vi "PR_Recording_post-processing.vi"(7 "Progress Bar Dialog in":refnum<class "Progress Bar Dialog.lvclass">, 8 "error in (no error)":errorcluster, 9 "Processing parameters":T2={"Defragment TDMS? (F)"=FALSE, "Start time (SW)"=timestamp(0 s since 1904-01-01), "Start time (HW)"=0, "Data filtering"={"Filter type"=enum."Savitzky-Golay", "Length"=41, "Order"=3}, "Mouse drawing parameters"={"Trace length, samples"=0, "Rainbow track"=FALSE, "Rainbow track is speed"=FALSE, "Bright mouse lineout"=FALSE, "Colors array"=[], "Pixels per mm"=0.0}, "Size of the image (480x480)"={"Numeric Control"=480.0, "Numeric Control"=480.0}, "Image ref. in"=refnum, "Calibration parameters"={"Timing calibration sw/hw"=1.0, "True FPS"=80.0, "True frame time, s"=0.0125, "Disp. calibration info"=[]}, "Pixel to zone"=[]} {"Calibration parameters"."True frame time, s" format="%.10g"; "Calibration parameters"."Disp. calibration info"."Speed, µl per ms" format="%.3g"; "Calibration parameters"."True FPS" format="%.10g"; "Calibration parameters"."Timing calibration sw/hw" format="%.10g"; "Data filtering"."Order" min=3 max=11 step=2; "Data filtering"."Length" min=5 max=301 step=2}, 10 "Paths":T9, 11 "Settings cluster":T10={"Defaults"={"Default User"=0.0, "VISA Resource Name "="", "Histogram parameters"={"max"=300.0, "min"=0.0, "# bins"=10, "threshold"=8.0, "thr. type"=enum."higher accepted"}}, "Recording and saving"={"Researcher name"="", "Name prefix"="", "Data post-processing"={"Filter type"=enum."None", "Length"=0, "Order"=0}, "Stop at"=0.0, "\"Stop at\" enabled"=FALSE, "Default save folder path"=path "", "Acquisition FPS"=enum."Max"}, "Geometry"={"Cage diameter, mm"=0, "Starting angle MIDFIELD"=0, "Starting angle BORDER"=0, "Radius, mm CENTER"=0, "Radius, mm MIDFIELD"=0, "N segments MIDFIELD"=0, "N segments BORDER"=0, "R-gap, mm"=0.0, "Bridge swap"=FALSE, "Bridge H. offset"=0.0, "Bridge V. offset"=0.0, "Twisted neck"=FALSE, "Alt. magn. orientation"=FALSE, "Sensor board size"=enum."Small"}, "IO parameters"={"IO general config."=0, "IO 1 configuration"=0, "IO 2 configuration"=0, "IO 3 configuration"=0, "IO 4 configuration"=0, "Activate ext. RS-232"=0, "IO inversion config."=0, "Sync capability"=0}, "Conditions presets array"=[], "Calibration parameters"={"Timing calibration sw/hw"=0.0, "True FPS"=0.0, "True frame time, s"=0.0, "Disp. calibration info"=[]}, "Settings loaded OK"=FALSE} {"Calibration parameters"."True frame time, s" format="%.10g"; "Calibration parameters"."Disp. calibration info"."Speed, µl per ms" format="%.3g"; "Calibration parameters"."True FPS" format="%.10g"; "Calibration parameters"."Timing calibration sw/hw" format="%.10g"; "Conditions presets array"."Specifier(s)"."Validity criteria(s)"."Validity value" min=0.0 step=0.1 format="%.2g"; "Conditions presets array"."Specifier(s)"."Value" step=1.0 format="%#.2g"; "Recording and saving"."Data post-processing"."Order" min=3 max=11 step=2; "Recording and saving"."Data post-processing"."Length" min=5 max=301 step=2; "Geometry"."Cage diameter, mm" scale=0.0..340.0}) -> (0 "error out":errorcluster, 2 "Loaded array data out":dbl[][](array[numeric]), 3 "Overlays cluster out":T1)   [LabVIEW 2018, in "Tracker.lvlib"]
uses:
  Tracker.lvlib
  Controls/CTL_Settings_cluster.ctl
  Controls/CTL_Histogram_parameters.ctl
  Controls/CTL_Filter_selector.ctl
  Controls/CTL_Acquisition_speed_selector.ctl
  Controls/CTL_Segmented_plot_parameters.ctl
  Controls/CTL_IO_params_cluster.ctl
  Controls/CTL_Conditions_Array.ctl
  Controls/CTL_Conditions_Cluster.ctl
  Controls/CTL_Condition_type.ctl
  Controls/CTL_Comparison_type.ctl
  Controls/CTL_Validity_check_criteria.ctl
  Controls/CTL_Response_info.ctl
  Controls/CTL_Condition_response_type.ctl
  Controls/CTL_Reponse_port_info.ctl
  Controls/CTL_Calibration_parameters.ctl
  Controls/CTL_Dispenser_calibration_info.ctl
  Controls/CTL_Paths_cluster.ctl
  <vilib>/ProgressBar/Progress Bar Dialog.lvclass
  Controls/CTL_Post-processing_params.ctl
  Controls/CTL_Mouse_Draw_Params.ctl
  <vilib>/vision/Image Controls.llb/IMAQ Image.ctl
  Controls/CTL_Pixel_to_Zone_array.ctl
  Controls/CTL_Overlays_cluster.ctl
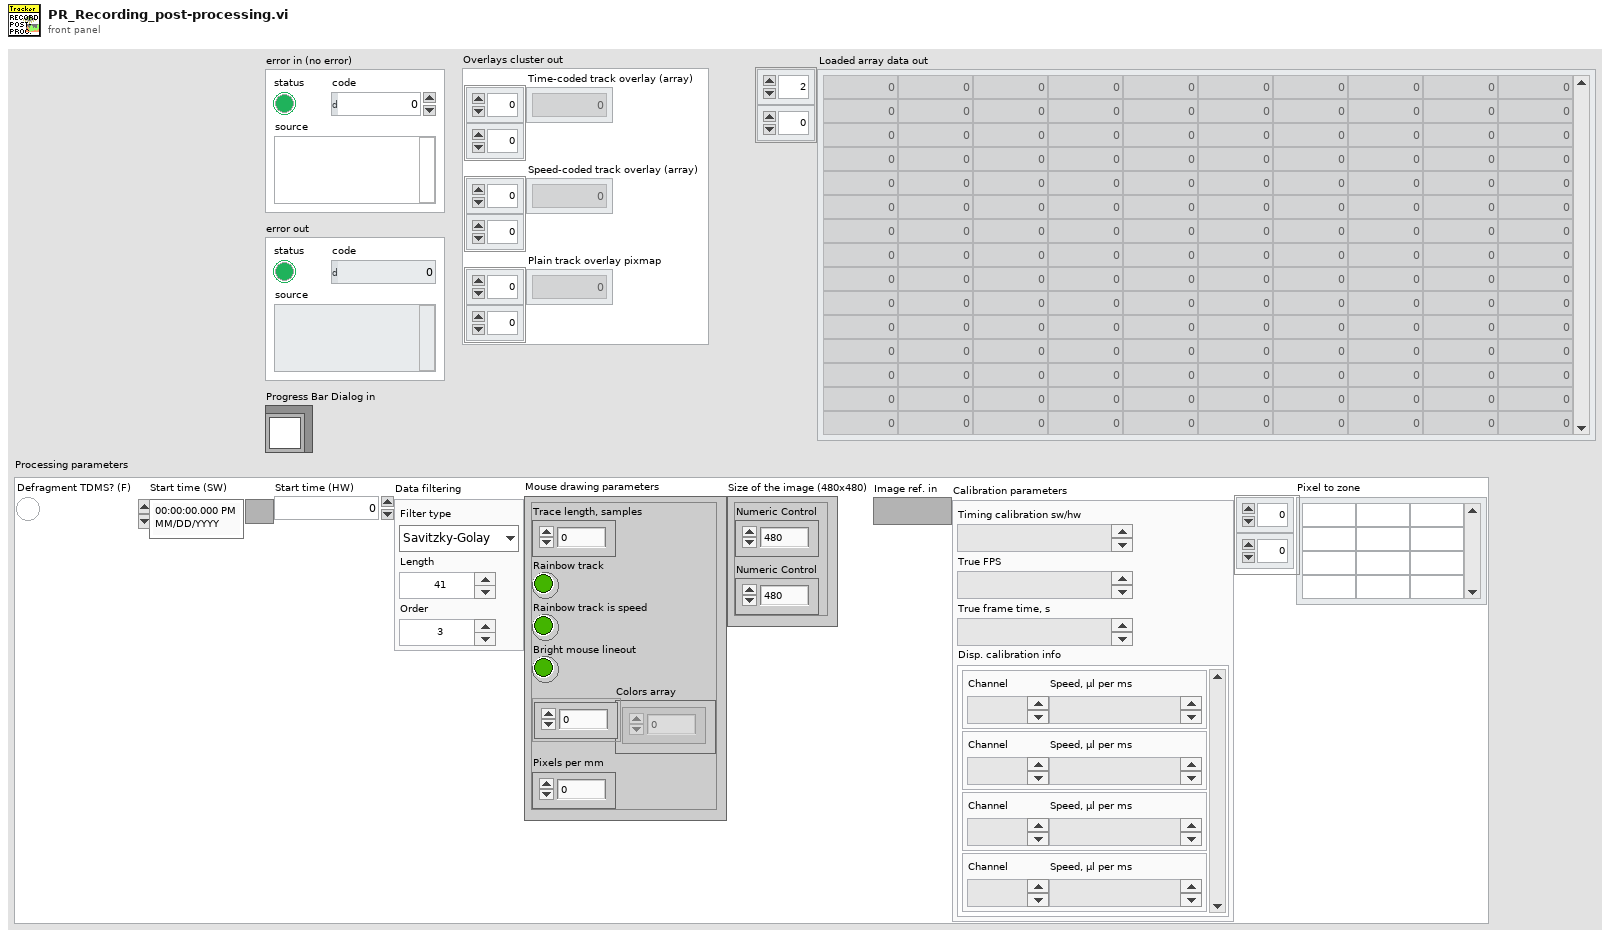
[diagram p1: front panel]
types:
  T1 = typedef "Tracker.lvlib/CTL_Overlays_cluster.ctl" = cluster{"Time-coded track overlay (array)":u32[][], "Speed-coded track overlay (array)":u32[][], "Plain track overlay pixmap":u32[][]}
  T2 = typedef "Tracker.lvlib/CTL_Post-processing_params.ctl" = cluster{"Defragment TDMS? (F)":bool, "Start time (SW)":timestamp, "Start time (HW)":u32, "Data filtering":T3, "Mouse drawing parameters":T4, "Size of the image (480x480)":cluster{"Numeric Control":dbl, "Numeric Control":dbl}, "Image ref. in":T5, "Calibration parameters":T6, "Pixel to zone":T8}
  T3 = typedef "Tracker.lvlib/CTL_Filter_selector.ctl" = cluster{"Filter type":enum16{"None", "Savitzky-Golay"}, "Length":i32, "Order":i32}
  T4 = typedef "Tracker.lvlib/CTL_Mouse_Draw_Params.ctl" = cluster{"Trace length, samples":u16, "Rainbow track":bool, "Rainbow track is speed":bool, "Bright mouse lineout":bool, "Colors array":u32[], "Pixels per mm":dbl}
  T5 = typedef "IMAQ Image.ctl" = refnum<image>
  T6 = typedef "Tracker.lvlib/CTL_Calibration_parameters.ctl" = cluster{"Timing calibration sw/hw":dbl, "True FPS":dbl, "True frame time, s":dbl, "Disp. calibration info":T7}
  T7 = typedef "Tracker.lvlib/CTL_Dispenser_calibration_info.ctl" = cluster{"Channel":u8, "Speed, µl per ms":dbl}[]
  T8 = typedef "Tracker.lvlib/CTL_Pixel_to_Zone_array.ctl" = i8[][]
  T9 = typedef "Tracker.lvlib/CTL_Paths_cluster.ctl" = cluster{"Program settings":path, "Folder":path, "TDMS file reference":refnum<k34>, "TDMS track":path, "Track settings":path, "Layout picture":path, "Density map matrix":path, "Density map picture":path, "ZIP":path}
  T10 = typedef "Tracker.lvlib/CTL_Settings_cluster.ctl" = cluster{"Defaults":cluster{"Default User":dbl, "VISA Resource Name ":string, "Histogram parameters":T11}, "Recording and saving":cluster{"Researcher name":string, "Name prefix":string, "Data post-processing":T3, "Stop at":dbl, "\"Stop at\" enabled":bool, "Default save folder path":path, "Acquisition FPS":T12}, "Geometry":T13, "IO parameters":T14, "Conditions presets array":T15, "Calibration parameters":T6, "Settings loaded OK":bool}
  T11 = typedef "Tracker.lvlib/CTL_Histogram_parameters.ctl" = cluster{"max":dbl, "min":dbl, "# bins":i32, "threshold":dbl, "thr. type":enum16{"higher accepted", "lower accepted"}}
  T12 = typedef "Tracker.lvlib/CTL_Acquisition_speed_selector.ctl" = enum16{"Max", "Optimal", "Eco"}
  T13 = typedef "Tracker.lvlib/CTL_Segmented_plot_parameters.ctl" = cluster{"Cage diameter, mm":u16, "Starting angle MIDFIELD":i16, "Starting angle BORDER":i16, "Radius, mm CENTER":u16, "Radius, mm MIDFIELD":u16, "N segments MIDFIELD":u8, "N segments BORDER":u8, "R-gap, mm":sgl, "Bridge swap":bool, "Bridge H. offset":sgl, "Bridge V. offset":sgl, "Twisted neck":bool, "Alt. magn. orientation":bool, "Sensor board size":enum16{"Small", "Large"}}
  T14 = typedef "Tracker.lvlib/CTL_IO_params_cluster.ctl" = cluster{"IO general config.":u16, "IO 1 configuration":u16, "IO 2 configuration":u16, "IO 3 configuration":u16, "IO 4 configuration":u16, "Activate ext. RS-232":u16, "IO inversion config.":u16, "Sync capability":u8}
  T15 = typedef "Tracker.lvlib/CTL_Conditions_Array.ctl" = T16[]
  T16 = typedef "Tracker.lvlib/CTL_Conditions_Cluster.ctl" = cluster{"Enabled":bool, "Name":string, "Specifier(s)":cluster{"Specifier enabled":bool, "Condition type":T17, "Comparison type":T18, "Value":dbl, "Validity criteria(s)":cluster{"V. check enabled":bool, "Criteria":T19, "Validity value":dbl}[]}[], "Response":T20, "Has been set":bool}
  T17 = typedef "Tracker.lvlib/CTL_Condition_type.ctl" = enum16{"Speed", "Zone", "Angle to wall"}
  T18 = typedef "Tracker.lvlib/CTL_Comparison_type.ctl" = enum16{"Less", "Less or Equal", "Equal", "Greater or Equal", "Greater", "Not Equal"}
  T19 = typedef "Tracker.lvlib/CTL_Validity_check_criteria.ctl" = enum16{"Running bout (seconds)", "Running bout (meters)"}
  T20 = typedef "Tracker.lvlib/CTL_Response_info.ctl" = cluster{"Response type":T21, "TTL port":T22, "TTL pulse length, ms":dbl}
  T21 = typedef "Tracker.lvlib/CTL_Condition_response_type.ctl" = enum16{"None", "Air puff", "Liquid reward"}
  T22 = typedef "Tracker.lvlib/CTL_Reponse_port_info.ctl" = enum16{"Port 1", "Port 2", "Port 3", "Port 4"}
  T23 = typedef "Tracker.lvlib/CTL_Cage_Coords_(arrays).ctl" = cluster{"R from center":dbl[], "sin(a)":dbl[], "Mouse Xc":dbl[], "Mouse Yc":dbl[], "X1-X2":dbl[], "Y1-Y2":dbl[], "Cage Xc":dbl[], "Cage Yc":dbl[], "Frame time, s":dbl}
  T24 = cluster{"Numeric Control":dbl, "Numeric Control":dbl}
  T25 = typedef "Tracker.lvlib/CTL_Animal_Coordinates_and_Speed_(arr).ctl" = cluster{"R from center":dbl[], "phi (mouse angular position in the cage)":dbl[], "alpha (mouse rot. angle)":dbl[], "X":dbl[], "Y":dbl[], "theta (from center towards mouse)":dbl[], "beta (cage rot. against mouse)":dbl[], "w (mouse angle to wall)":dbl[], "Speed (filtered)":dbl[], "Zone":i8[]}
  T26 = cluster{"Boolean Round":bool, "code":i32, "source":string}
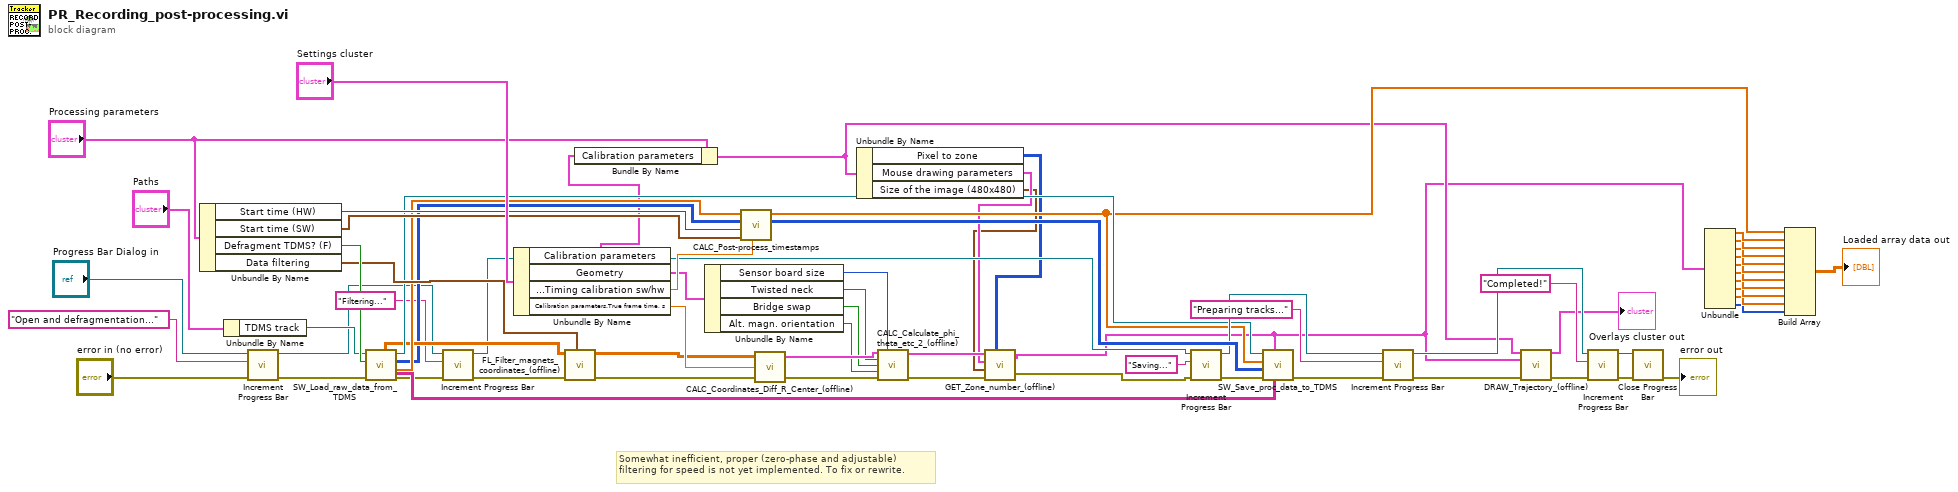
[diagram p0: block diagram]
diagram:
  # "Somewhat inefficient, proper (zero-phase and adjustable) filtering for speed is not yet implemented. To fix or rewrite."
  n1 = Unbundle By Name("Processing parameters") -> ("Start time (HW)"=w42:u32, "Start time (SW)"=w41:timestamp, "Defragment TDMS? (F)"=w44:bool, "Data filtering"=w43:T3)
  n2 = Unbundle By Name("Paths") -> ("TDMS track"=w33:path)
  n3 = call <vilib>:"Increment Progress Bar.vi"("error in (no error)"="error in (no error)", "Step Name (\"\")"="Open and defragmentation..." ("Step Name (\"\")"), "Progress Bar Dialog in"="Progress Bar Dialog in") -> ("error out"=w60:errorcluster, "Progress Bar Dialog out"=w24:refnum<class "Progress Bar Dialog.lvclass">)  [unwired: 6 in, 1 out]
  n4 = call "SW_Load_raw_data_from_TDMS.vi"("error in (no error)"=w60, "Defragment TDMS? (F)"=w44, "TDMS track ref. in"=w33) -> ("error out"=w27:errorcluster, "SW timestamp"=w31:dbl[], "HW ts and Frame HW time"=w28:u32[][], "TDMS track ref. out"=w32:refnum<k34>, "TTL IO and Key"=w30:string[][], "Raw values"=w29:dbl[][])  [unwired: 3 in]
  n5 = call <vilib>:"Increment Progress Bar.vi"("error in (no error)"=w27, "Step Name (\"\")"="Filtering..." ("Step Name (\"\")"), "Progress Bar Dialog in"=w24) -> ("error out"=w26:errorcluster, "Progress Bar Dialog out"=w23:refnum<class "Progress Bar Dialog.lvclass">)  [unwired: 6 in, 1 out]
  n6 = Unbundle By Name("Settings cluster") -> ("Calibration parameters"=w22:T6, "Geometry"=w49:T13, "Calibration parameters.Timing calibration sw/hw"=w65:dbl, "Calibration parameters.True frame time, s"=w63:dbl)
  n7 = call "FL_Filter_magnets_coordinates_(offline).vi"("Data filtering"=w43, "error in (no error)"=w26, "Magnets raw coordinates in"=w29) -> ("error out"=w64:errorcluster, "Magnets filtered coordinates out"=w62:dbl[][])  [unwired: 7 in]
  n8 = Bundle By Name(cluster="Processing parameters", "Calibration parameters"=w22) -> (w10:T2)
  n9 = Unbundle By Name(w49) -> ("Sensor board size"=w45:enum16{"Small", "Large"}, "Twisted neck"=w48:bool, "Bridge swap"=w47:bool, "Alt. magn. orientation"=w46:bool)
  n10 = call "CALC_Post-process_timestamps.vi"("Timing calibration sw/hw"=w65, "Start time (SW)"=w41, "Start time (HW)"=w42, "HW timestamp and delta in"=w28, "SW timestamp in"=w31) -> ("HW timestamp and delta out"=w66:u32[][], "SW timestamp out"=w11:dbl[])  [unwired: 5 in]
  n11 = call "CALC_Coordinates_Diff_R_Center_(offline).vi"("Error In"=w64, "Frame time, s"=w63, "Magnets coordinates in"=w62) -> ("Error Out"=w51:errorcluster, "Output cluster of data"=w50:T23)  [unwired: 1 in]
  n12 = Unbundle By Name(w10) -> ("Pixel to zone"=w2:T8, "Mouse drawing parameters"=w5:T4, "Size of the image (480x480)"=w4:T24)
  n13 = call "CALC_Calculate_phi_theta_etc_2_(offline).vi"("Input data cluster"=w50, "SB size"=w45, "Twisted neck"=w48, "Bridge swap"=w47, "Use alternative magnets orientation"=w46, "Error In"=w51) -> ("Animal coordinates cluster"=w6:T25, "Error out"=w9:errorcluster)  [unwired: 8 in]
  n14 = call "GET_Zone_number_(offline).vi"("Animal coordinates cluster in"=w6, "Mouse drawing parameters"=w5, "Size of the image (480x480)"=w4, "error in (no error)"=w9, "Array of the pixel to zone correspondences"=w2) -> ("Animal coordinates cluster out"=w7:T25, "error out"=w8:T26)
  n15 = call <vilib>:"Increment Progress Bar.vi"("error in (no error)"=w8, "Step Name (\"\")"="Saving..." ("Step Name (\"\")"), "Progress Bar Dialog in"=w23) -> ("error out"=w52:errorcluster, "Progress Bar Dialog out"=w36:refnum<class "Progress Bar Dialog.lvclass">)  [unwired: 6 in, 1 out]
  n16 = call "SW_Save_proc_data_to_TDMS.vi"("TTL IO and Key in"=w30, "Processed animal coordinates and speed"=w7, "error in (no error)"=w52, "HW timestamp and delta in"=w66, "SW timestamp in"=w11, "TDMS file ref. in"=w32) -> ("error out"=w38:errorcluster)  [unwired: 5 in]
  n17 = call <vilib>:"Increment Progress Bar.vi"("error in (no error)"=w38, "Step Name (\"\")"="Preparing tracks..." ("Step Name (\"\")"), "Progress Bar Dialog in"=w36) -> ("error out"=w37:errorcluster, "Progress Bar Dialog out"=w35:refnum<class "Progress Bar Dialog.lvclass">)  [unwired: 6 in, 1 out]
  n18 = call "DRAW_Trajectory_(offline).vi"("Processing parameters"=w10, "Animal coordinates and speed"=w7, "Error In"=w37) -> ("Overlays cluster out"=→"Overlays cluster out":T1, "Error Out"=w39:errorcluster)  [unwired: 11 in]
  n19 = call <vilib>:"Increment Progress Bar.vi"("error in (no error)"=w39, "Step Name (\"\")"="Completed!" ("Step Name (\"\")"), "Progress Bar Dialog in"=w35) -> ("error out"=w53:errorcluster, "Progress Bar Dialog out"=w54:refnum<class "Progress Bar Dialog.lvclass">)  [unwired: 6 in, 1 out]
  n20 = call <vilib>:"Close Progress Bar.vi"("error in (no error)"=w53, "Progress Bar Dialog"=w54) -> ("error out"=→"error out":errorcluster)  [unwired: 9 in]
  n21 = Unbundle(w7) -> ("R from center"=w21:dbl[], "phi (mouse angular position in the cage)"=w20:dbl[], "alpha (mouse rot. angle)"=w19:dbl[], "X"=w18:dbl[], "Y"=w17:dbl[], "theta (from center towards mouse)"=w16:dbl[], "beta (cage rot. against mouse)"=w15:dbl[], "w (mouse angle to wall)"=w14:dbl[], "Speed (filtered)"=w13:dbl[], "Zone"=w3:i8[])
  n22 = Build Array(w11, w21, w20, w19, w18, w17, w16, w15, w14, w13, w3) -> (→"Loaded array data out":dbl[][])
